vi "GET_G_EQUIP_COMM.vi"() -> (3 "G_EQUIP_CMM":T1)   [LabVIEW 2018]
uses:
  G_EQUIP_CMM.vi
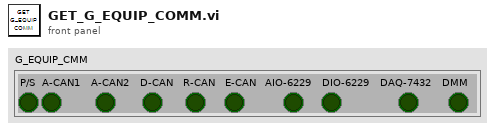
[diagram p1: front panel]
types:
  T1 = cluster{"P/S":bool, "A-CAN1":bool, "A-CAN2":bool, "D-CAN":bool, "R-CAN":bool, "E-CAN":bool, "AIO-6229":bool, "DIO-6229":bool, "DAQ-7432":bool, "DMM":bool}
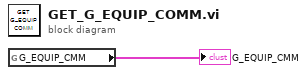
[diagram p0: block diagram]
diagram:
  n1 = global read "G_EQUIP_CMM.vi" "G_EQUIP_CMM"() -> (→"G_EQUIP_CMM":T1)
